vi "Week1_Slide38_SineWave.vi"() -> ()   [LabVIEW 2015]
panel:
  in  "Phase":dbl
  in  "Frequency in Hz":dbl
  out "Iteration":i32
  in  "stop":bool
  out "Waveform Chart":dbl(graph)
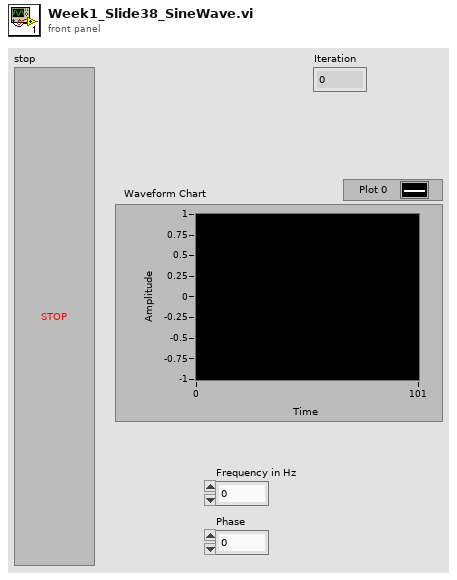
[diagram p1: front panel]
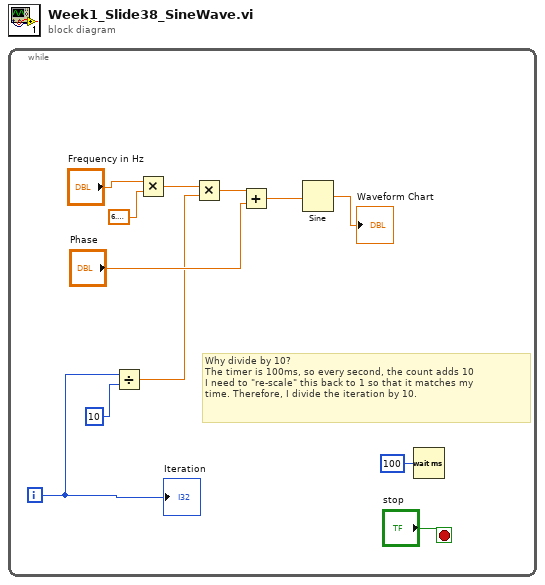
[diagram p0: block diagram]
diagram:
  n1 = while {
    i -> [w5]
    stop <- "stop" stop-if-true
    # "Why divide by 10? \nThe timer is 100ms, so every second, the count adds 10\nI need to \"re-scale\" this back to 1 so that it matches my\ntime. Therefore, I divide the iteration by 10."
    n2 = Divide(x=w5, y=10) -> (x/y=w4:dbl)
    n3 = Multiply(x="Frequency in Hz", y=6.283185307179586) -> (x*y=w2:dbl)
    n4 = Multiply(x=w2, y=w4) -> (x*y=w10:dbl)
    n5 = Add(x=w10, y="Phase") -> (x+y=w8:dbl)
    n6 = Sine(x=w8) -> (sin(x)=→"Waveform Chart":dbl)
    n7 = Wait (ms)(milliseconds to wait=u32 100) -> ()  [unwired: 1 out]
    "Iteration" <- w5
  }
